vi "Get library description.vi"(11 "Library in":refnum<vi>) -> (0 "error out":errorcluster, 3 "Description":string)   [LabVIEW 2019, in "Panther Dashboard.lvlib"]
uses:
  Panther Dashboard.lvlib
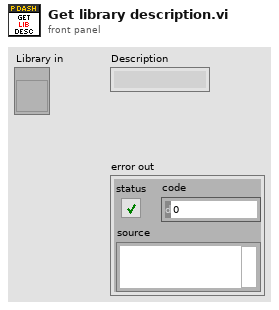
[diagram p1: front panel]
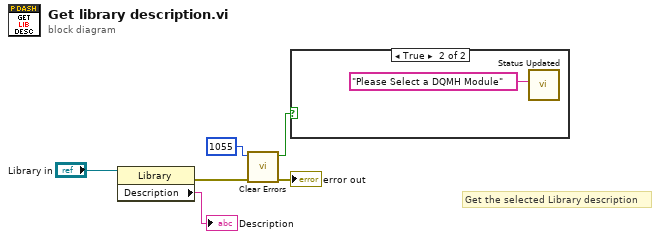
[diagram p0: block diagram]
diagram:
  # "Get the selected Library description"
  n1 = property class="Library"(reference="Library in") -> (error out=w5:errorcluster, "Description"=→"Description":string)  [unwired: 1 in, 1 out]
  n2 = call <vilib>:"Clear Errors.vi"("error in (no error)"=w5, "specific error code to clear (0: all)"=1055) -> ("error out"=→"error out":errorcluster, "specific error cleared?"=w4:bool)  [unwired: 4 in]
  n3 = case shown="True" w4 {
    frame False {
    }
    frame True {
      n4 = call "Status Updated.vi"("Status"="Please Select a DQMH Module") -> ()  [unwired: 10 in, 1 out]
    }
  }
